vi "Rectangle Contains Point (ltrb).vi"(4 "Point":cluster{"x":dbl, "y":dbl}, 5 "Rectangle":T1) -> (1 "Contained?":bool)   [LabVIEW 2020]
uses:
  Graphics VIs/Rectangle (double).ctl
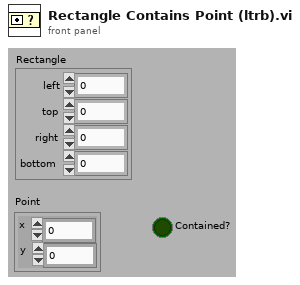
[diagram p1: front panel]
types:
  T1 = typedef "Rectangle (double).ctl" = cluster{"left":dbl, "top":dbl, "right":dbl, "bottom":dbl}
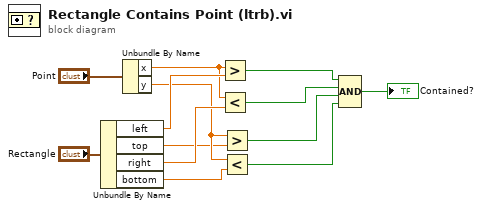
[diagram p0: block diagram]
diagram:
  n1 = Unbundle By Name("Rectangle") -> ("left"=w11:dbl, "top"=w6:dbl, "right"=w9:dbl, "bottom"=w7:dbl)
  n2 = Unbundle By Name("Point") -> ("x"=w10:dbl, "y"=w8:dbl)
  n3 = Greater?(x=w10, y=w11) -> (0:w5:bool)
  n4 = Less?(x=w10, y=w9) -> (x < y?=w4:bool)
  n5 = Greater?(x=w8, y=w6) -> (0:w3:bool)
  n6 = Less?(x=w8, y=w7) -> (x < y?=w2:bool)
  n7 = Compound Arithmetic op=AND(w5, w4, w3, w2) -> (→"Contained?":bool)
